vi "Get Attribute Meta Data.vi"(7 "Unique ID":string, 8 "error in (no error)":errorcluster, 9 "Attribute Type":variant, 10 "Attribute Name":string, 11 "Test Executive in":refnum<class "Test Executive.lvclass">) -> (0 "error out":errorcluster, 1 "Found?":bool, 2 "Meta Data":string, 3 "Test Executive out":refnum<class "Test Executive.lvclass">)   [LabVIEW 2017, in "Test Executive.lvlib" / "Test Executive.lvclass"]
uses:
  <vilib>/gpm_packages/@cs/test-executive/Source/Test Executive/TestExecutive/Test Executive.lvclass
  <vilib>/gpm_packages/@cs/test-executive/Source/Test Executive/TestExecutive/Test Executive.lvclass/Test Executive.ctl
  <vilib>/gpm_packages/@cs/linked-list/Source/Linked List/Linked List Ref/Linked List Ref.lvclass
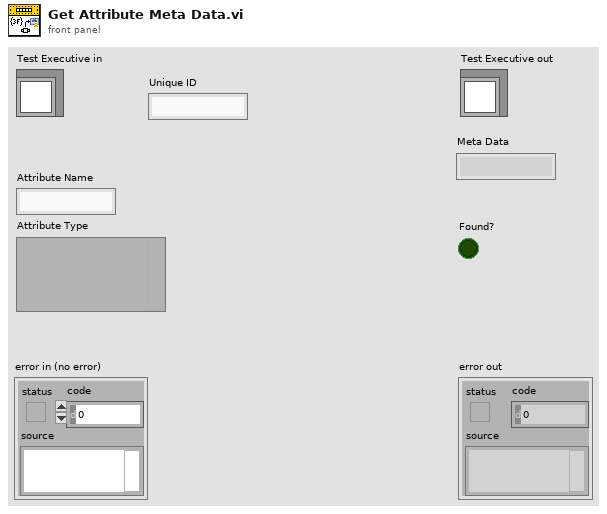
[diagram p1: front panel]
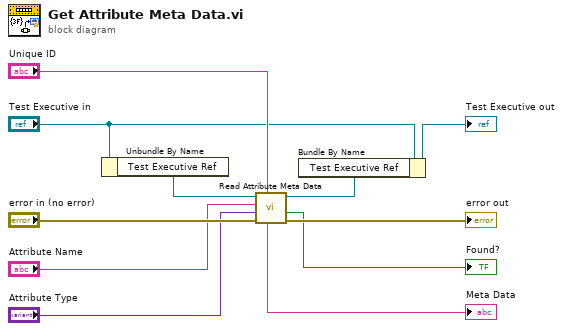
[diagram p0: block diagram]
diagram:
  n1 = Unbundle By Name("Test Executive in") -> ("Test Executive Ref"=w4:refnum<data-value>)
  n2 = call <vilib>:"Read Attribute Meta Data.vi"("Linked List ID"="Unique ID", "error in (no error)"="error in (no error)", "Attribute Type"="Attribute Type", "Attribute Name"="Attribute Name", "Linked List Ref"=w4) -> ("error out"=→"error out":errorcluster, "Found?"=→"Found?":bool, "Linked List Ref out"=w3:refnum<data-value>, "Meta Data"=→"Meta Data":string)  [unwired: 3 in]
  n3 = Bundle By Name(cluster="Test Executive in", "Test Executive Ref"=w3) -> (→"Test Executive out":refnum<class "Test Executive.lvclass">)
